vi "3channel.vi"() -> ()   [LabVIEW 2014]
doc: "Personal Daq 54 example.\nTriggering is immediate and readings are returned 1 scan at a time as available.\nBe sure to use the Acquisition Stop control for proper shutdown."
uses:
  <vilib>/Utility/error.llb/DialogType.ctl
  <vilib>/DAQmx/read.llb/DAQmx Read (Analog 1D DBL NChan 1Samp).vi
  <vilib>/Analysis/2dsp.llb/Complex FFT.vi
  <vilib>/DAQmx/create/channels.llb/DAQmx Create Channel (AI-Voltage-Basic).vi
  <vilib>/DAQmx/configure/timing.llb/DAQmx Timing (Sample Clock).vi
  <vilib>/DAQmx/miscellaneous.llb/DAQmx Fill In Error Info.vi
  <vilib>/measure/madcrms.llb/Basic Averaged DC-RMS for 1 Chan.vi
  Instance           2 26Saved   noise_Nov07_2009_5 .vi
  Instance          18 26Saved   noise_Nov07_2009_5 .vi
  <vilib>/express/express analysis/Spectral/Block/exnSpectralBlock spectral measurements peak poly.vi
  <vilib>/express/express analysis/Spectral/Block/exnSpectralBlock spectral measurements peak DDT.vi
  Instance           1 26Saved   noise_Nov07_2009_5 .vi
  Instance           4 26Saved   noise_Nov07_2009_5 .vi
  <vilib>/express/express analysis/Spectral/XNode/ExpressSpectralMeasurementsBlockNode.xnode
  <vilib>/measure/NI_MAPro.lvlib
  <vilib>/Analysis/NI_AALPro.lvlib
panel:
  out "I/Q Signal 2":waveform(dbl)(graph)
  in  "Save Data":bool
  in  "Max. Heartrate":i32=90
  in  "Min. Heartrate":i32=50
  out "Heartrate":dbl
  out "max value 2":dbl
  in  "Max. Resp. Rate":i32=30
  in  "Min. Resp. Rate":i32=10
  out "Resp. Rate":dbl
  out "max value":dbl
  out "Record":dynamicdata(graph)
  in  "input terminal configuration":i32(ring)=10083 items=["default"=-1, "RSE"=10083, "NRSE"=10078, "Differential"=10106, "Pseudodifferential"=12529]
  out "error out":errorcluster
  in  "stop":bool
  in  "Maximum Value":dbl=5.0 format="%0.2f"
  in  "Minimum Value":dbl=-2.0 format="%0.2f"
  in  "Rate":dbl=20.0 caption="Sample Rate (Hz)" format="%0.2f"
  in  "Samples per Channel":i32=1
  out "Combined Spectrum":waveform(dbl)(graph)
  out "I/Q Spectrum":dynamicdata(graph)
  out "Respiration Q":dbl=19.665142208058892 format="%#_3g"
  out "Respiration I":dbl=19.7 format="%#_3g"
  in  "FFT":i32=256
  out "I/Q Signal":dynamicdata(graph)
  in  "t0":timestamp=timestamp(3198752888.296 s since 1904-01-01)
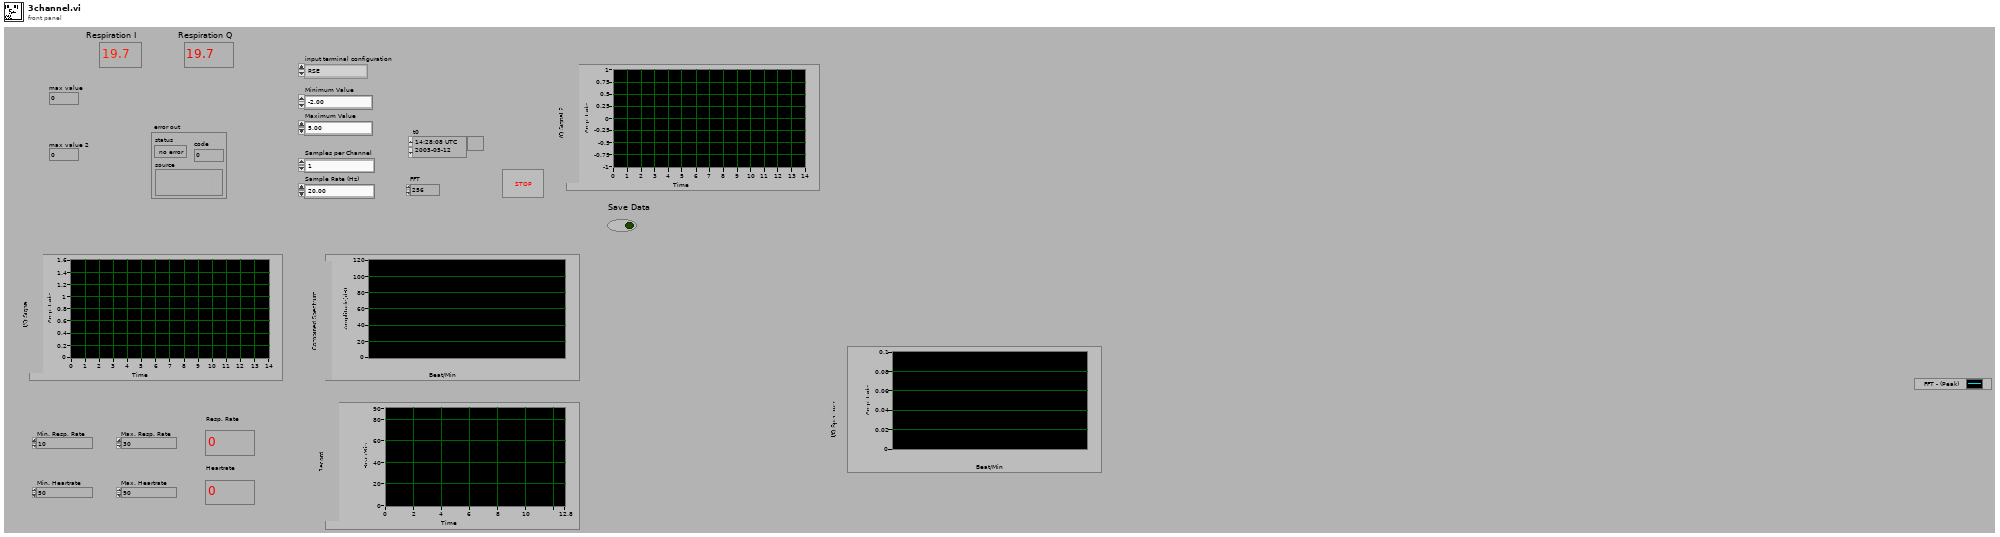
[diagram p1: front panel]
types:
  T1 = typedef "DialogType.ctl" = u16
  T2 = cluster{"averaging mode":u16, "weighting mode":u16, "number of averages":u32}
  T3 = cluster{"dB On (F)":bool, "unwrap phase (F)":bool, "convert to degree (F)":bool}
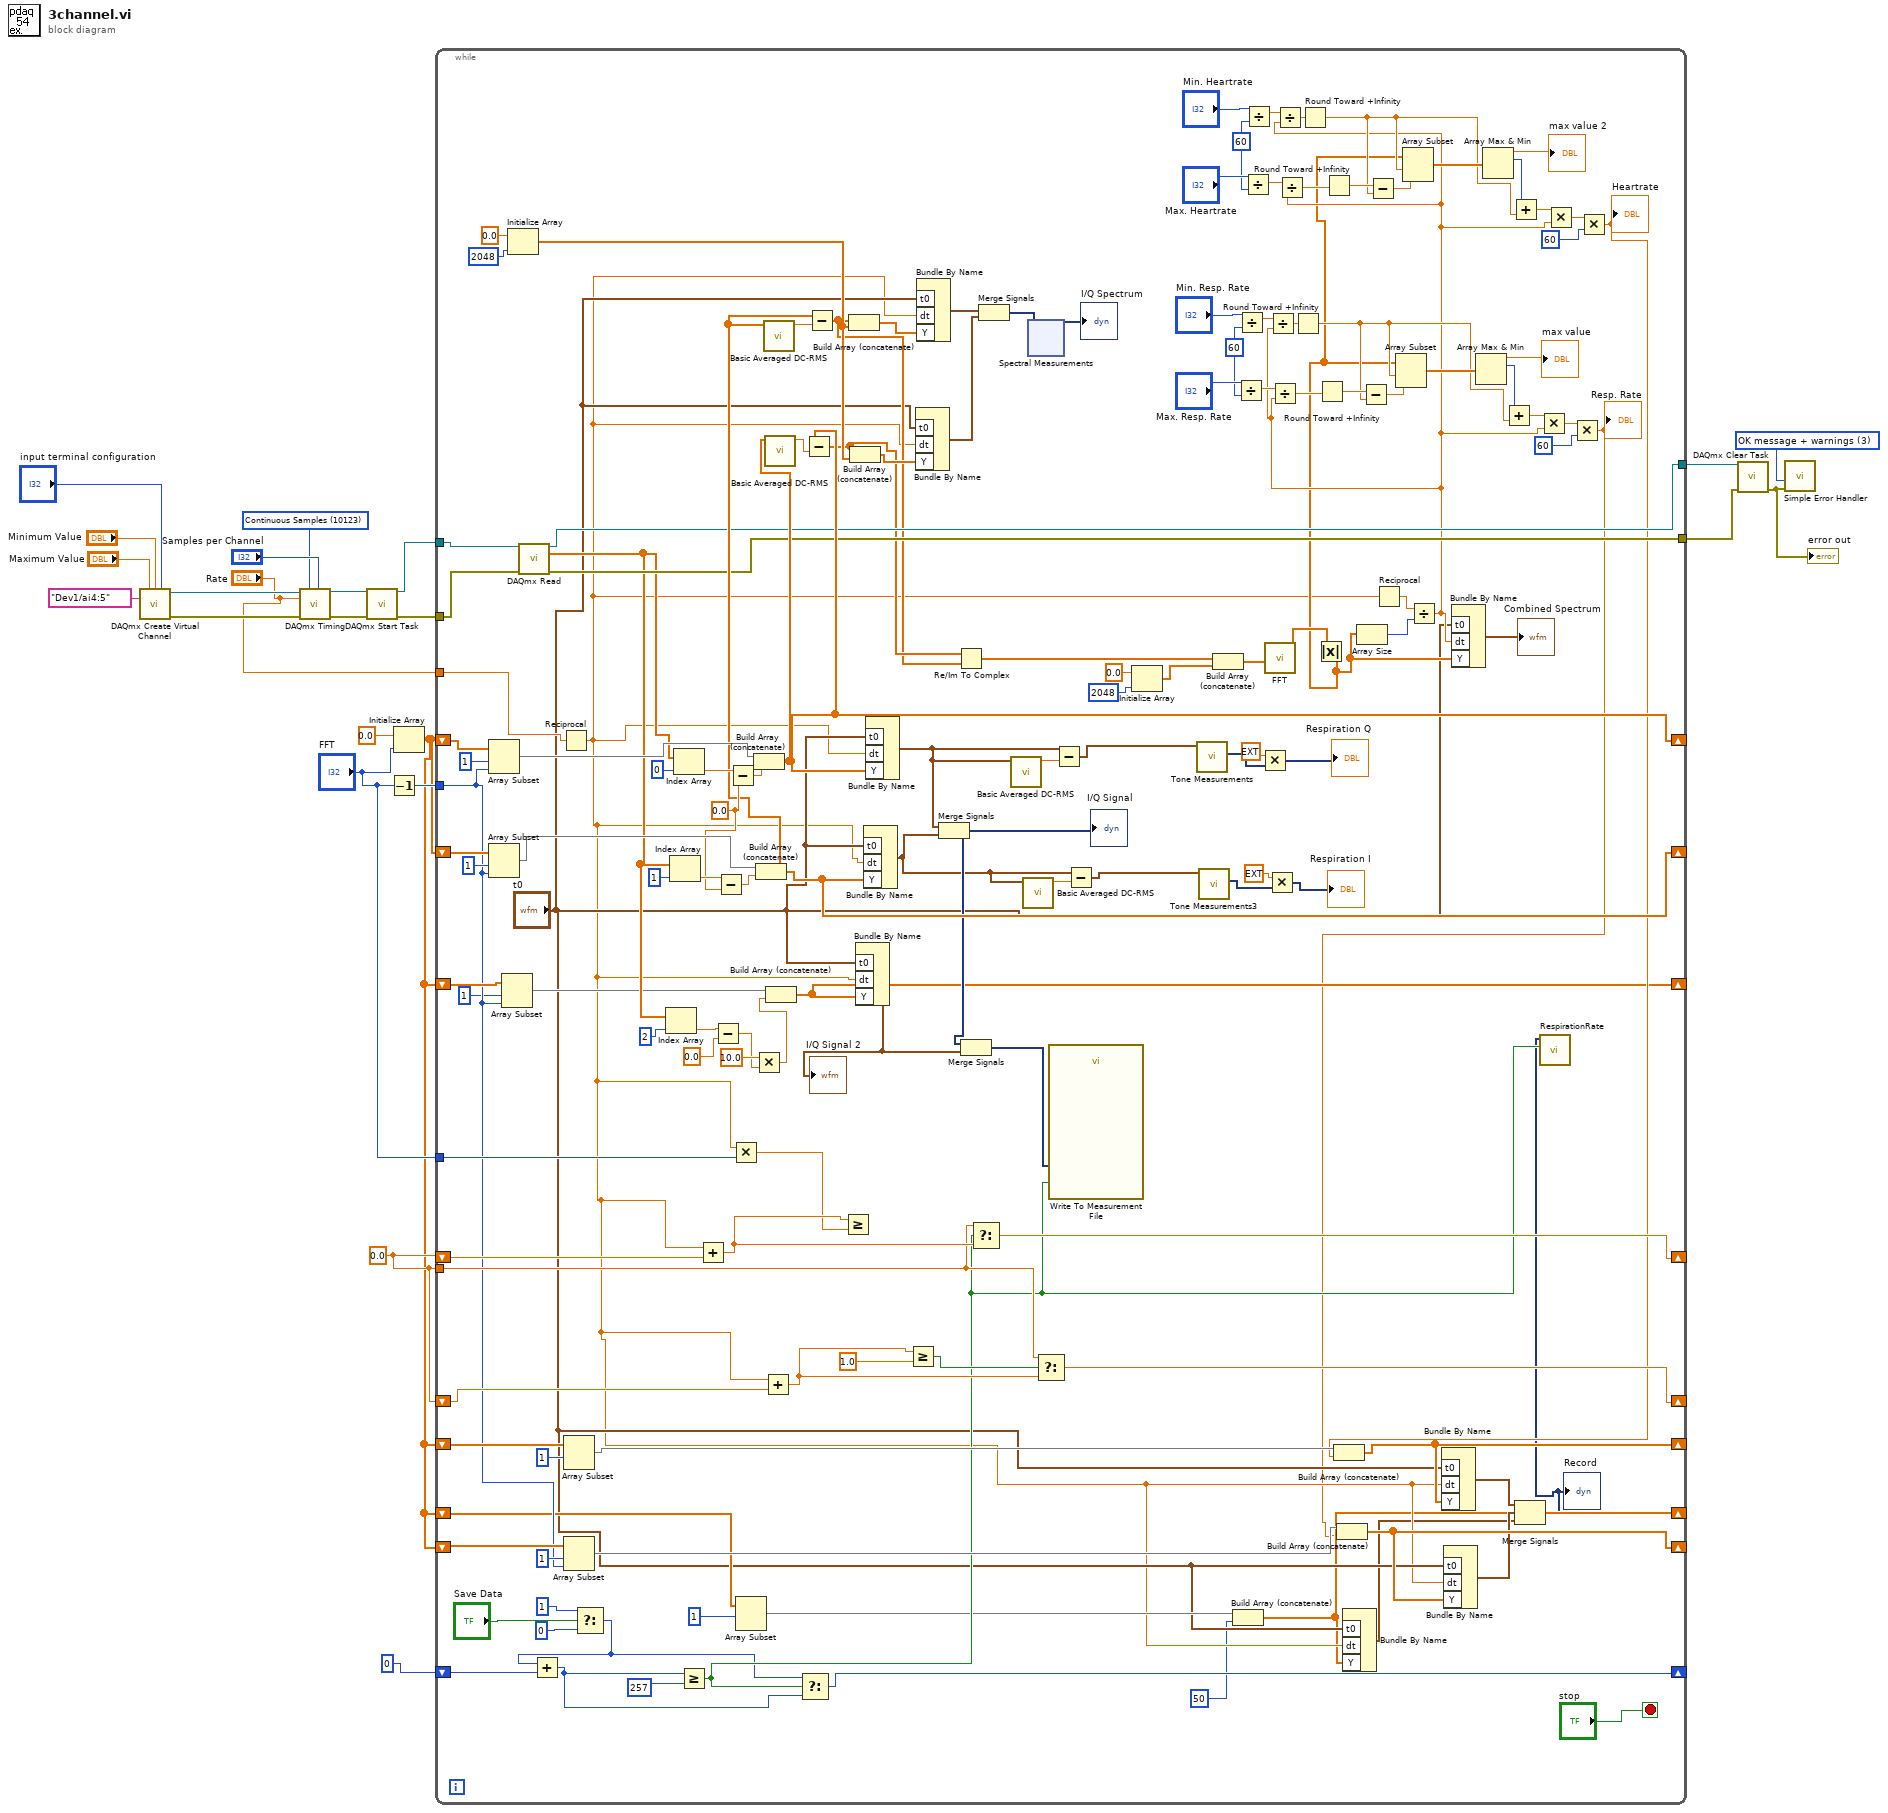
[diagram p0: block diagram]
diagram:
  w3 = 0.0 ("element")
  w9 = T1 3 items=["no dialog", "OK message", "continue or stop message", "OK message + warnings", "continue/stop + warnings"] ("type of dialog (OK msg:1)")
  w16 = 10123 items=["Finite Samples"=10178, "Continuous Samples"=10123] ("sample mode")
  n1 = call-poly <vilib>:"DAQmx Create Virtual Channel.vi"("maximum value"="Maximum Value", "minimum value"="Minimum Value", "input terminal configuration"="input terminal configuration", "physical channels"=tag "Dev1/ai4:5") -> ("task out"=w17:refnum<k21>, "error out"=w19:errorcluster)  [unwired: 5 in, 5 out]
  n2 = call-poly <vilib>:"DAQmx Timing.vi"("task/channels in"=w17, "sample mode"=w16, "samples per channel"="Samples per Channel", "rate"="Rate", "error in"=w19) -> ("task out"=w15:refnum<k21>, "error out"=w14:errorcluster)  [unwired: 2 in, 7 out]
  n3 = call <vilib>:"DAQmx Start Task.vi"("task/channels in"=w15, "error in"=w14) -> ("task out"=w12:refnum<k21>, "error out"=w11:errorcluster)  [unwired: 12 out]
  n4 = Decrement(x="FFT") -> (x-1=w22:i32)
  n5 = Initialize Array(0.0 ("element"), "FFT") -> (w1:dbl[])
  n6 = while {
    shift-right: [w135] -> _
    shift-left: w1 -> [w167]
    tunnel: w22 -> [w46]
    shift-right: [w134] -> _
    shift-left: w1 -> [w158]
    tunnel: w12 -> [w133]
    tunnel: w11 -> [w132]
    tunnel: "Rate" -> [w131]
    tunnel: [w130] -> w8
    tunnel: [w129] -> w7
    shift-right: [w121] -> _
    shift-left: w3 -> [w118]
    tunnel: "FFT" -> [w120]
    tunnel: w3 -> [w112]
    shift-right: [w116] -> _
    shift-left: w3 -> [w113]
    shift-right: [w96] -> _
    shift-left: w1 -> [w104]
    shift-right: [w97] -> _
    shift-left: w1 -> [w100]
    shift-right: [w54] -> _
    shift-left: 0 -> [w57]
    shift-right: [w39] -> _
    shift-left: w1 -> [w47]
    shift-right: [w32] -> _
    shift-left: w1 -> [w38]
    stop <- "stop" stop-if-true
    w60 = 60
    w76 = 60
    w152 = 0.0 ("element")
    n7 = Array Subset(array=w167, index=1, length=w46) -> (w165:dbl[])
    n8 = Array Subset(array=w158, index=1, length=w46) -> (w156:dbl[])
    n9 = Array Subset(array=w47, index=1, length=w46) -> (w40:dbl[])
    n10 = Initialize Array(0.0 ("element"), 2048 ("dimension size")) -> (w126:dbl[])
    n11 = call-poly <vilib>:"DAQmx Read.vi"("task/channels in"=w133, "error in"=w132) -> ("task out"=w130:refnum<k21>, "data"=w43:dbl[], "error out"=w129:errorcluster)  [unwired: 11 out]
    n12 = Reciprocal(x=w131) -> (1/x=w34:dbl)
    n13 = Array Subset(array=w100, index=1) -> (w99:dbl[])  [unwired: 1 in]
    n14 = Array Subset(array=w104, index=1, length=w46) -> (w103:dbl[])
    n15 = Select(t=1, s="Save Data", f=0) -> (s? t:f=w50:i32)
    n16 = Add(x=w50, y=w57) -> (x+y=w55:i32)
    n17 = Index Array(array=w43, index=2 ("index (row)")) -> (element=w42:dbl)
    n18 = Index Array(array=w43, index=1 ("index (row)")) -> (element=w153:dbl)
    n19 = Index Array(array=w43, index=0 ("index (row)")) -> (element=w154:dbl)
    n20 = Greater Or Equal?(x=w55, y=257) -> (x >= y?=w53:bool)
    n21 = Add(x=w34, y=w118) -> (x+y=w122:dbl)
    n22 = Subtract(x=w42, y=0.0 ("element")) -> (x-y=w27:dbl)
    n23 = Subtract(x=w153, y=w152) -> (x-y=w145:dbl)
    n24 = Subtract(x=w154, y=w152) -> (x-y=w146:dbl)
    n25 = Multiply(x=w34, y=w120) -> (x*y=w119:dbl)
    n26 = Array Subset(array=w38, index=1) -> (w36:dbl[])  [unwired: 1 in]
    n27 = Build Array (concatenate)(w165, w146) -> (w135:dbl[])
    n28 = Multiply(x=10.0, y=w27) -> (x*y=w26:dbl)
    n29 = Build Array (concatenate)(w156, w145) -> (w134:dbl[])
    n30 = Add(x=w34, y=w113) -> (x+y=w117:dbl)
    n31 = call-poly <vilib>:"Basic Averaged DC-RMS.vi"("signal in"=w134) -> ("DC value"=w144:dbl)  [unwired: 4 in, 6 out]
    n32 = call-poly <vilib>:"Basic Averaged DC-RMS.vi"("signal in"=w135) -> ("DC value"=w143:dbl)  [unwired: 4 in, 6 out]
    n33 = Build Array (concatenate)(w40, w26) -> (w39:dbl[])
    n34 = Select(t=w50, s=w53, f=w55) -> (s? t:f=w54:i32)
    n35 = Subtract(x=w135, y=w143) -> (x-y=w124:dbl[])
    n36 = Subtract(x=w134, y=w144) -> (x-y=w123:dbl[])
    n37 = Greater Or Equal?(x=w122, y=w119) -> ()  [unwired: 1 out]
    n38 = Build Array (concatenate)(w123, w126) -> (w150:dbl[])
    n39 = Build Array (concatenate)(w124, w126) -> (w151:dbl[])
    n40 = Bundle By Name("t0"="t0", "dt"=w34, "Y"=w39) -> (w24:waveform(dbl))  [unwired: 1 out]
    "I/Q Signal 2" <- w24
    n41 = Bundle By Name("t0"="t0", "dt"=w34, "Y"=w134) -> (w106:waveform(dbl))  [unwired: 1 out]
    n42 = Bundle By Name("t0"="t0", "dt"=w34, "Y"=w135) -> (w109:waveform(dbl))  [unwired: 1 out]
    n43 = Greater Or Equal?(x=w117, y=1.0) -> (x >= y?=w114:bool)
    n44 = Bundle By Name("t0"="t0", "dt"=w34, "Y"=w151) -> (w140:waveform(dbl))  [unwired: 1 out]
    n45 = Bundle By Name("t0"="t0", "dt"=w34, "Y"=w150) -> (w141:waveform(dbl))  [unwired: 1 out]
    n46 = Merge Signals(w109, w106) -> (w125:dynamicdata)
    "I/Q Signal" <- w125
    n47 = Re/Im To Complex(1:w123, 2:w124) -> (0:w147:cdb[])
    n48 = Merge Signals(w125, w24) -> (w25:dynamicdata)
    n49 = Select(t=w112, s=w53, f=w122) -> (s? t:f=w121:dbl)
    n50 = Merge Signals(w141, w140) -> (w142:dynamicdata)
    n51 = call-poly <vilib>:"Basic Averaged DC-RMS.vi"("signal in"=w109) -> ("DC value"=w111:dbl)  [unwired: 4 in, 6 out]
    n52 = call-poly <vilib>:"Basic Averaged DC-RMS.vi"("signal in"=w106) -> ("DC value"=w108:dbl)  [unwired: 4 in, 6 out]
    n53 = xnode "Spectral Measurements"("Signals"=w142) -> ("FFT - (Peak)"=→"I/Q Spectrum":dynamicdata)  [unwired: 2 in, 3 out]
    n54 = Select(t=w112, s=w114, f=w117) -> (s? t:f=w116:dbl)
    n55 = call "Write To Measurement File"("Signals"=w25, "Enable"=w53) -> ()  [unwired: 5 in, 13 out]
    n56 = Subtract(x=w109, y=w111) -> (x-y=w110:waveform(dbl))
    n57 = Subtract(x=w106, y=w108) -> (x-y=w107:waveform(dbl))
    n58 = Initialize Array(0.0 ("element"), 2048 ("dimension size")) -> (w148:dbl[])
    n59 = call "Tone Measurements"("Signals"=w110) -> ("Frequency"=w162:dynamicdata)  [unwired: 1 in, 9 out]
    n60 = call "Tone Measurements3"("Signals"=w107) -> ("Frequency"=w159:dynamicdata)  [unwired: 1 in, 9 out]
    n61 = Build Array (concatenate)(w147, w148) -> (w136:cdb[])
    n62 = Build Array (concatenate)(w36, 50 ("index")) -> (w32:dbl[])
    n63 = Divide(x="Max. Resp. Rate", y=w76) -> (x/y=w91:dbl)
    n64 = Divide(x="Min. Resp. Rate", y=w76) -> (x/y=w92:dbl)
    n65 = Divide(x="Max. Heartrate", y=w60) -> (x/y=w74:dbl)
    n66 = Divide(x="Min. Heartrate", y=w60) -> (x/y=w75:dbl)
    n67 = Multiply(x=ext 60.0, y=w162) -> (x*y=→"Respiration Q":dynamicdata)
    n68 = call-poly <vilib>:"FFT.vi"("X"=w136) -> ("FFT {X}"=w139:cdb[])  [unwired: 2 in, 8 out]
    n69 = Multiply(x=ext 60.0, y=w159) -> (x*y=→"Respiration I":dynamicdata)
    n70 = Absolute Value(x=w139) -> (abs(x)=w48:dbl[])
    n71 = Bundle By Name("t0"="t0", "dt"=w34, "Y"=w32) -> (w33:waveform(dbl))  [unwired: 1 out]
    n72 = Array Size(array=w48) -> (size(s)=w137:i32)
    n73 = Reciprocal(x=w34) -> (1/x=w79:dbl)
    n74 = Divide(x=w79, y=w137) -> (x/y=w59:dbl)
    n75 = Divide(x=w92, y=w59) -> (x/y=w90:dbl)
    n76 = Divide(x=w91, y=w59) -> (x/y=w89:dbl)
    n77 = Divide(x=w75, y=w59) -> (x/y=w73:dbl)
    n78 = Divide(x=w74, y=w59) -> (x/y=w72:dbl)
    n79 = Round Toward +Infinity(x=w90) -> (ceil(x): smallest int >= x=w83:dbl)
    n80 = Round Toward +Infinity(x=w73) -> (ceil(x): smallest int >= x=w66:dbl)
    n81 = Round Toward +Infinity(x=w89) -> (ceil(x): smallest int >= x=w87:dbl)
    n82 = Round Toward +Infinity(x=w72) -> (ceil(x): smallest int >= x=w70:dbl)
    n83 = Subtract(x=w87, y=w83) -> (x-y=w88:dbl)
    n84 = Subtract(x=w70, y=w66) -> (x-y=w71:dbl)
    n85 = Array Subset(array=w48, index=w83, length=w88) -> (w86:dbl[])
    n86 = Array Subset(array=w48, index=w66, length=w71) -> (w69:dbl[])
    n87 = Bundle By Name("t0"="t0", "dt"=w59, "Y"=w48) -> (→"Combined Spectrum":waveform(dbl))  [unwired: 1 out]
    n88 = Array Max & Min(array=w86) -> (max value=→"max value":dbl, max index (indices)=w84:i32)  [unwired: 2 out]
    n89 = Array Max & Min(array=w69) -> (max value=→"max value 2":dbl, max index (indices)=w67:i32)  [unwired: 2 out]
    n90 = Add(x=w84, y=w83) -> (x+y=w82:dbl)
    n91 = Add(x=w67, y=w66) -> (x+y=w65:dbl)
    n92 = Multiply(x=w82, y=w59) -> (x*y=w81:dbl)
    n93 = Multiply(x=w65, y=w59) -> (x*y=w64:dbl)
    n94 = Multiply(x=w81, y=60) -> (x*y=w30:dbl)
    "Resp. Rate" <- w30
    n95 = Build Array (concatenate)(w103, w30) -> (w96:dbl[])
    n96 = Bundle By Name("t0"="t0", "dt"=w34, "Y"=w96) -> (w94:waveform(dbl))  [unwired: 1 out]
    n97 = Multiply(x=w64, y=60) -> (x*y=w58:dbl)
    "Heartrate" <- w58
    n98 = Build Array (concatenate)(w99, w58) -> (w97:dbl[])
    n99 = Bundle By Name("t0"="t0", "dt"=w34, "Y"=w97) -> (w95:waveform(dbl))  [unwired: 1 out]
    n100 = Merge Signals(w95, w94, w33) -> (w31:dynamicdata)
    "Record" <- w31
    n101 = call "RespirationRate"("Enable"=w53, "Signals"=w31) -> ()  [unwired: 3 in, 7 out]
  }
  n102 = call <vilib>:"DAQmx Clear Task.vi"("task in"=w8, "error in"=w7) -> ("error out"=w6:errorcluster)  [unwired: 13 out]
  "error out" <- w6
  n103 = call <vilib>:"Simple Error Handler.vi"("type of dialog (OK msg:1)"=w9, "error in (no error)"=w6) -> ()  [unwired: 8 out]
